vi "SineWaverTangoInterfaceManager.vi"(0 "?":bool, 1 "Instance Name":string="1", 2 "Executable Name":string="LabviewSingleDeviceDServer") -> ()   [LabVIEW 2014, in "examples.lvlib"]
uses:
  examples.lvlib
  vis/tango_vi.llb/_DServerClientRequest.ctl
  vis/tango_vi.llb/_DServerClientRequestType.ctl
  vis/tango_vi.llb/_DServerClientRequestData.ctl
  vis/tango_vi.llb/_GenericDataBuffer.ctl
  vis/tango_vi.llb/_AttributeDataType_t.ctl
  vis/tango_vi.llb/_TangoState_t.ctl
  sinewavercontrols.vi
  vis/tango_vi.llb/_DServerSetStateScalarAttributeValue.vi
  vis/tango_vi.llb/_DServerSetStringScalarAttributeValue.vi
  vis/tango_vi.llb/_DServerSetDoubleScalarAttributeValue.vi
  vis/tango_vi.llb/_DServerSetBooleanScalarAttributeValue.vi
  vis/tango_vi.llb/_DServerSetDoubleSpectrumAttributeValue.vi
  vis/tango_vi.llb/_DServerRequestDataToDoubleScalar.vi
  vis/tango_vi.llb/_DServerRequestDataToBooleanScalar.vi
  vis/tango_vi.llb/tango.lvlib
panel:
  out "Device List":string[](array[string])
  out "Client Request":T1={"Request Id"=0, "Source Id"=0, "Request Type"=enum."UNKNOWN_REQUEST", "Device Class Name"="unspecified_class_name", "Device Name"="unspecified/device/name", "Cmd or Attr Name"="unspecified_cmd_or_attr_name", "Client Request Data"={"write attribute value"={"dimx"=0, "dimy"=0, "data"=[], "data_type"=enum."UNKNOWN_DATA_TYPE"}, "exec. command argin"={"num data"=[], "str data"=[]}}}
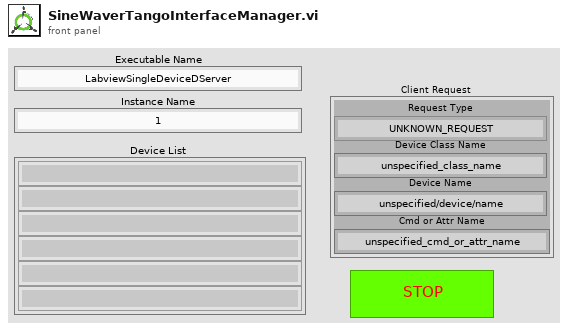
[diagram p1: front panel]
types:
  T1 = typedef "tango.lvlib/_DServerClientRequest.ctl" = cluster{"Request Id":u32, "Source Id":u32, "Request Type":T2, "Device Class Name":string, "Device Name":string, "Cmd or Attr Name":string, "Client Request Data":T3}
  T2 = typedef "tango.lvlib/_DServerClientRequestType.ctl" = enum16{"EXEC_CMD", "READ_ATTR", "WRITE_ATTR", "UNKNOWN_REQUEST"}
  T3 = typedef "tango.lvlib/_DServerClientRequestData.ctl" = cluster{"write attribute value":T4, "exec. command argin":cluster{"num data":u8[], "str data":string[]}}
  T4 = typedef "tango.lvlib/_GenericDataBuffer.ctl" = cluster{"dimx":u32, "dimy":u32, "data":u8[], "data_type":T5}
  T5 = typedef "tango.lvlib/_AttributeDataType_t.ctl" = enum16{"STATE_SCA", "STATE_SPE", "STATE_IMG", "STRING_SCA", "STRING_SPE", "STRING_IMG", "BOOL_SCA", "BOOL_SPE", "BOOL_IMG", "UCHAR_SCA", "UCHAR_SPE", "UCHAR_IMG", "SHORT_SCA", "SHORT_SPE", "SHORT_IMG", "USHORT_SCA", "USHORT_SPE", "USHORT_IMG", "LONG_SCA", "LONG_SPE", "LONG_IMG", "ULONG_SCA", "ULONG_SPE", "ULONG_IMG", "LONG64_SCA", "LONG64_SPE", "LONG64_IMG", "ULONG64_SCA", "ULONG64_SPE", "ULONG64_IMG", "FLOAT_SCA", "FLOAT_SPE", "FLOAT_IMG", "DOUBLE_SCA", "DOUBLE_SPE", "DOUBLE_IMG", "ENUM_SCA", "UNKNOWN_DATA_TYPE"}
  T6 = typedef "tango.lvlib/_DServerEvent.ctl" = cluster{"event registration refnum":refnum<event-registration>, "user event out":refnum<user-event>}
  T7 = typedef "tango.lvlib/_TangoState_t.ctl" = enum32{"ON", "OFF", "CLOSE", "OPEN", "INSERT", "EXTRACT", "MOVING", "STANDBY", "FAULT", "INIT", "RUNNING", "ALARM", "DISABLE", "UNKNOWN"}
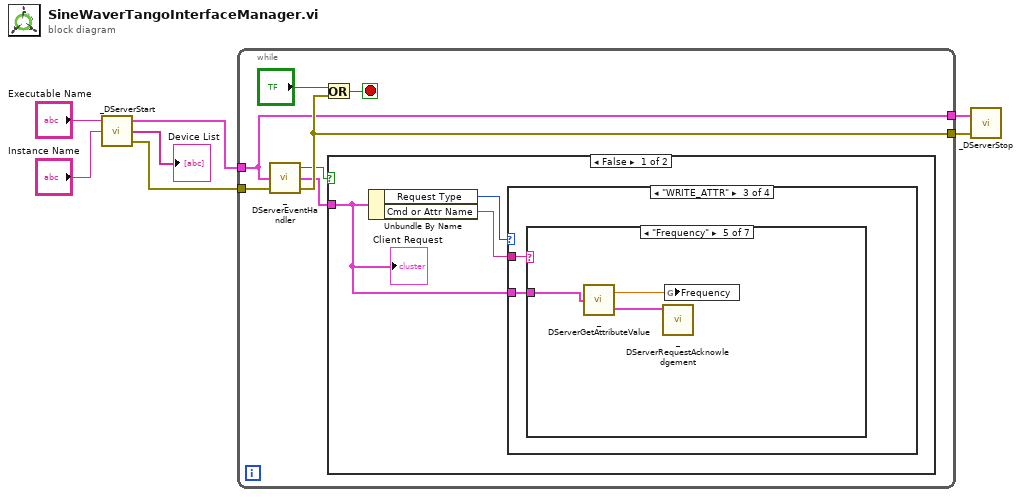
[diagram p0: block diagram]
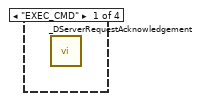
[diagram p2: hidden frame]
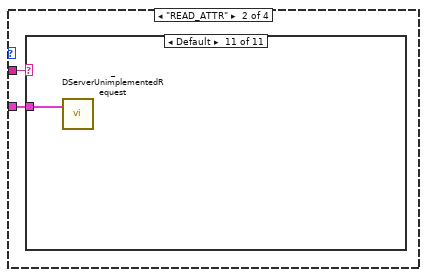
[diagram p3: hidden frame]
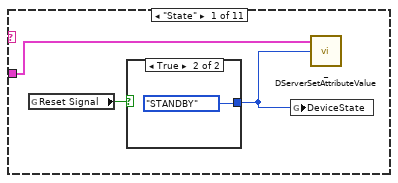
[diagram p4: hidden frame]
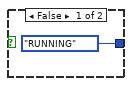
[diagram p5: hidden frame]
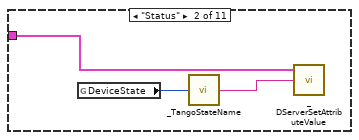
[diagram p6: hidden frame]
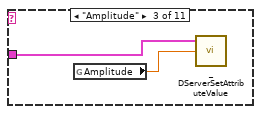
[diagram p7: hidden frame]
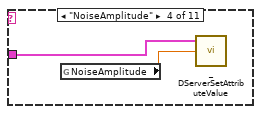
[diagram p8: hidden frame]
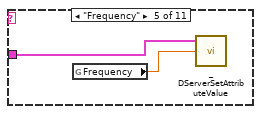
[diagram p9: hidden frame]
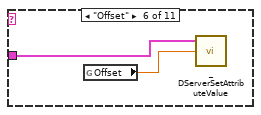
[diagram p10: hidden frame]
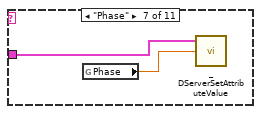
[diagram p11: hidden frame]
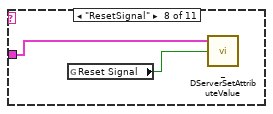
[diagram p12: hidden frame]
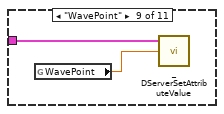
[diagram p13: hidden frame]
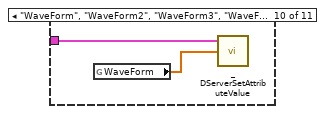
[diagram p14: hidden frame]
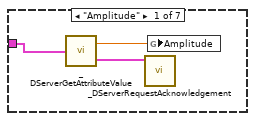
[diagram p15: hidden frame]
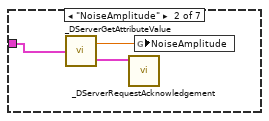
[diagram p16: hidden frame]
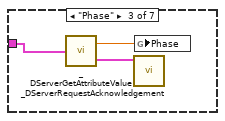
[diagram p17: hidden frame]
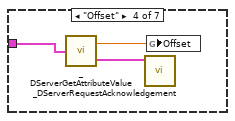
[diagram p18: hidden frame]
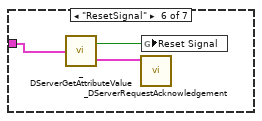
[diagram p19: hidden frame]
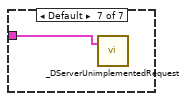
[diagram p20: hidden frame]
diagram:
  n1 = call "_DServerStart.vi"("instance name"="Instance Name", "executable name"="Executable Name") -> ("error out"=w7:errorcluster, "device_list"=→"Device List":string[], "dserver evt."=w3:T6)  [unwired: 1 in]
  n2 = while {
    tunnel: w7 -> [w13]
    tunnel: w3 -> [w11]
    tunnel: [w12] -> w2
    tunnel: [w11] -> w1
    stop <- w10 stop-if-true
    n3 = call "_DServerEventHandler.vi"("error in"=w13, "dserver evt."=w11) -> ("error out"=w12:errorcluster, "client request"=w9:T1, "timeout"=w8:bool)  [unwired: 1 in]
    n4 = Or(x="?", y=w12) -> (x .or. y?=w10:bool)
    n5 = case shown="False" w8 {
      tunnel: w9 -> [w15 _]
      frame False {
        n6 = Unbundle By Name(w15) -> ("Request Type"=w16:T2, "Cmd or Attr Name"=w17:string)
        n7 = case shown="\"WRITE_ATTR\"" w16 {
          tunnel: w17 -> [_ w19 w46 _]
          tunnel: w15 -> [_ w18 w45 _]
          frame "EXEC_CMD" {
            n8 = call "_DServerRequestAcknowledgement.vi"() -> ()  [unwired: 7 in, 1 out]
          }
          frame "READ_ATTR" {
            n9 = case shown="Default" w19 {
              tunnel: w18 -> [w20 w25 w28 w30 w32 w34 w36 w38 w41 w42 w44]
              frame "State" {
                n10 = global read "sinewavercontrols.vi" "Reset Signal"() -> (w22:bool)
                n11 = case shown="True" w22 {
                  tunnel: [_TangoState_t."RUNNING" ("Tango Device State") _TangoState_t."STANDBY" ("Tango Device State")] -> w21
                  frame False {
                  }
                  frame True {
                  }
                }
                n12 = global write "sinewavercontrols.vi" "DeviceState"(w21) -> ()
                n13 = call-poly "_DServerSetAttributeValue.vi"("value"=w21, "client request"=w20) -> ()  [unwired: 3 in, 1 out]
              }
              frame "Status" {
                n14 = global read "sinewavercontrols.vi" "DeviceState"() -> (w26:T7)
                n15 = call "_TangoStateName.vi"("State"=w26) -> ("State Name"=w27:string)
                n16 = call-poly "_DServerSetAttributeValue.vi"("value"=w27, "client request"=w25) -> ()  [unwired: 3 in, 1 out]
              }
              frame "Amplitude" {
                n17 = global read "sinewavercontrols.vi" "Amplitude"() -> (w29:dbl)
                n18 = call-poly "_DServerSetAttributeValue.vi"("value"=w29, "client request"=w28) -> ()  [unwired: 3 in, 1 out]
              }
              frame "NoiseAmplitude" {
                n19 = global read "sinewavercontrols.vi" "NoiseAmplitude"() -> (w31:dbl)
                n20 = call-poly "_DServerSetAttributeValue.vi"("value"=w31, "client request"=w30) -> ()  [unwired: 3 in, 1 out]
              }
              frame "Frequency" {
                n21 = global read "sinewavercontrols.vi" "Frequency"() -> (w33:dbl)
                n22 = call-poly "_DServerSetAttributeValue.vi"("value"=w33, "client request"=w32) -> ()  [unwired: 3 in, 1 out]
              }
              frame "Offset" {
                n23 = global read "sinewavercontrols.vi" "Offset"() -> (w35:dbl)
                n24 = call-poly "_DServerSetAttributeValue.vi"("value"=w35, "client request"=w34) -> ()  [unwired: 3 in, 1 out]
              }
              frame "Phase" {
                n25 = global read "sinewavercontrols.vi" "Phase"() -> (w37:dbl)
                n26 = call-poly "_DServerSetAttributeValue.vi"("value"=w37, "client request"=w36) -> ()  [unwired: 3 in, 1 out]
              }
              frame "ResetSignal" {
                n27 = global read "sinewavercontrols.vi" "Reset Signal"() -> (w39:bool)
                n28 = call-poly "_DServerSetAttributeValue.vi"(4:w39, "client request"=w38) -> ()  [unwired: 3 in, 1 out]
              }
              frame "WavePoint" {
                n29 = global read "sinewavercontrols.vi" "WavePoint"() -> (w40:dbl)
                n30 = call-poly "_DServerSetAttributeValue.vi"("value"=w40, "client request"=w41) -> ()  [unwired: 3 in, 1 out]
              }
              frame "WaveForm", "WaveForm2", "WaveForm3", "WaveForm4" {
                n31 = global read "sinewavercontrols.vi" "WaveForm"() -> (w43:dbl[])
                n32 = call-poly "_DServerSetAttributeValue.vi"("value"=w43, "client request"=w42) -> ()  [unwired: 3 in, 1 out]
              }
              frame Default {
                n33 = call "_DServerUnimplementedRequest.vi"("client request"=w44) -> ()  [unwired: 2 in, 1 out]
              }
            }
          }
          frame "WRITE_ATTR" {
            n34 = case shown="\"Frequency\"" w46 {
              tunnel: w45 -> [w47 w50 w53 w56 w59 w62 w65]
              frame "Amplitude" {
                n35 = call-poly "_DServerGetAttributeValue.vi"("client request"=w47) -> ("attribute value"=w49:dbl, "client request"=w48:T1)
                n36 = call "_DServerRequestAcknowledgement.vi"("client request"=w48) -> ()  [unwired: 6 in, 1 out]
                n37 = global write "sinewavercontrols.vi" "Amplitude"(w49) -> ()
              }
              frame "NoiseAmplitude" {
                n38 = call-poly "_DServerGetAttributeValue.vi"("client request"=w50) -> ("attribute value"=w52:dbl, "client request"=w51:T1)
                n39 = call "_DServerRequestAcknowledgement.vi"("client request"=w51) -> ()  [unwired: 6 in, 1 out]
                n40 = global write "sinewavercontrols.vi" "NoiseAmplitude"(w52) -> ()
              }
              frame "Phase" {
                n41 = call-poly "_DServerGetAttributeValue.vi"("client request"=w53) -> ("attribute value"=w55:dbl, "client request"=w54:T1)
                n42 = call "_DServerRequestAcknowledgement.vi"("client request"=w54) -> ()  [unwired: 6 in, 1 out]
                n43 = global write "sinewavercontrols.vi" "Phase"(w55) -> ()
              }
              frame "Offset" {
                n44 = call-poly "_DServerGetAttributeValue.vi"("client request"=w56) -> ("attribute value"=w58:dbl, "client request"=w57:T1)
                n45 = call "_DServerRequestAcknowledgement.vi"("client request"=w57) -> ()  [unwired: 6 in, 1 out]
                n46 = global write "sinewavercontrols.vi" "Offset"(w58) -> ()
              }
              frame "Frequency" {
                n47 = call-poly "_DServerGetAttributeValue.vi"("client request"=w59) -> ("attribute value"=w61:dbl, "client request"=w60:T1)
                n48 = call "_DServerRequestAcknowledgement.vi"("client request"=w60) -> ()  [unwired: 6 in, 1 out]
                n49 = global write "sinewavercontrols.vi" "Frequency"(w61) -> ()
              }
              frame "ResetSignal" {
                n50 = call-poly "_DServerGetAttributeValue.vi"("client request"=w62) -> ("attribute value"=w64:bool, "client request"=w63:T1)
                n51 = call "_DServerRequestAcknowledgement.vi"("client request"=w63) -> ()  [unwired: 6 in, 1 out]
                n52 = global write "sinewavercontrols.vi" "Reset Signal"(w64) -> ()
              }
              frame Default {
                n53 = call "_DServerUnimplementedRequest.vi"("client request"=w65) -> ()  [unwired: 2 in, 1 out]
              }
            }
          }
          frame "UNKNOWN_REQUEST", Default {
            n54 = call "_DServerUnimplementedRequest.vi"() -> ()  [unwired: 3 in, 1 out]
          }
        }
        "Client Request" <- w15
      }
      frame True {
      }
    }
  }
  n55 = call "_DServerStop.vi"("error in"=w2, "dserver evt."=w1) -> ()  [unwired: 1 in, 1 out]
